vi "DriveToDistance.vi"() -> (0 "Drive Y Command":dbl format="%#_13g", 3 "Drive X Command":dbl format="%#_13g")   [LabVIEW 2016]
uses:
  Robot Global Data.vi
  <vilib>/addons/control/pid/pid.llb/PID Lead-Lag (DBL).vi
  <vilib>/addons/control/pid/pid.llb/PID (DBL).vi
  <vilib>/addons/control/pid/NI_PID_pid.lvlib
panel:
  in  "PID gains":T1={"proportional gain (Kc)"=0.05, "integral time (Ti, min)"=0.0, "derivative time (Td, min)"=0.0} {"derivative time (Td, min)" format="%.3f"; "integral time (Ti, min)" format="%.3f"; "proportional gain (Kc)" format="%.3f"}
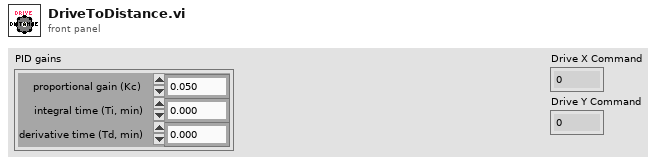
[diagram p1: front panel]
types:
  T1 = cluster{"proportional gain (Kc)":dbl, "integral time (Ti, min)":dbl, "derivative time (Td, min)":dbl}
  T2 = enum16{"FL Drive Wheel", "FR Drive Wheel", "RL Drive Wheel", "RR Drive Wheel", "FL Steer Wheel", "FR Steer Wheel", "RL Steer Wheel", "RR Steer Wheel"}
  T3 = typedef "WPI_MotorControlDeviceRef.ctl" = cluster{"DeviceStatus":errorcluster, "Type":T4, "PWM":cluster{"PWM Channel":T5, "DeadBand":T6}, "CAN":cluster{"Device Number":u8, "SetOutput VI Ref":variant, "GetOutput VI Ref":variant, "Enable VI Ref":variant, "Disable VI Ref":variant, "Data":variant}, "Invert":bool}
  T4 = typedef "WPI_MotorControlType.ctl" = enum16{"PWM", "CAN"}
  T5 = typedef "FPGA_DIOPWMChannel.ctl" = enum8{"PWM 0", "PWM 1", "PWM 2", "PWM 3", "PWM 4", "PWM 5", "PWM 6", "PWM 7", "PWM 8", "PWM 9", "PWM MXP 0", "PWM MXP 1", "PWM MXP 2", "PWM MXP 3", "PWM MXP 4", "PWM MXP 5", "PWM MXP 6", "PWM MXP 7", "PWM MXP 8", "PWM MXP 9", "Invalid"}
  T6 = typedef "WPI_PWMDeadband.ctl" = cluster{"Name":string, "maxPositivePwm":i32, "minPositivePwm":i32, "centerPwm":i32, "maxNegativePwm":i32, "minNegativePwm":i32, "angularRange":u16}
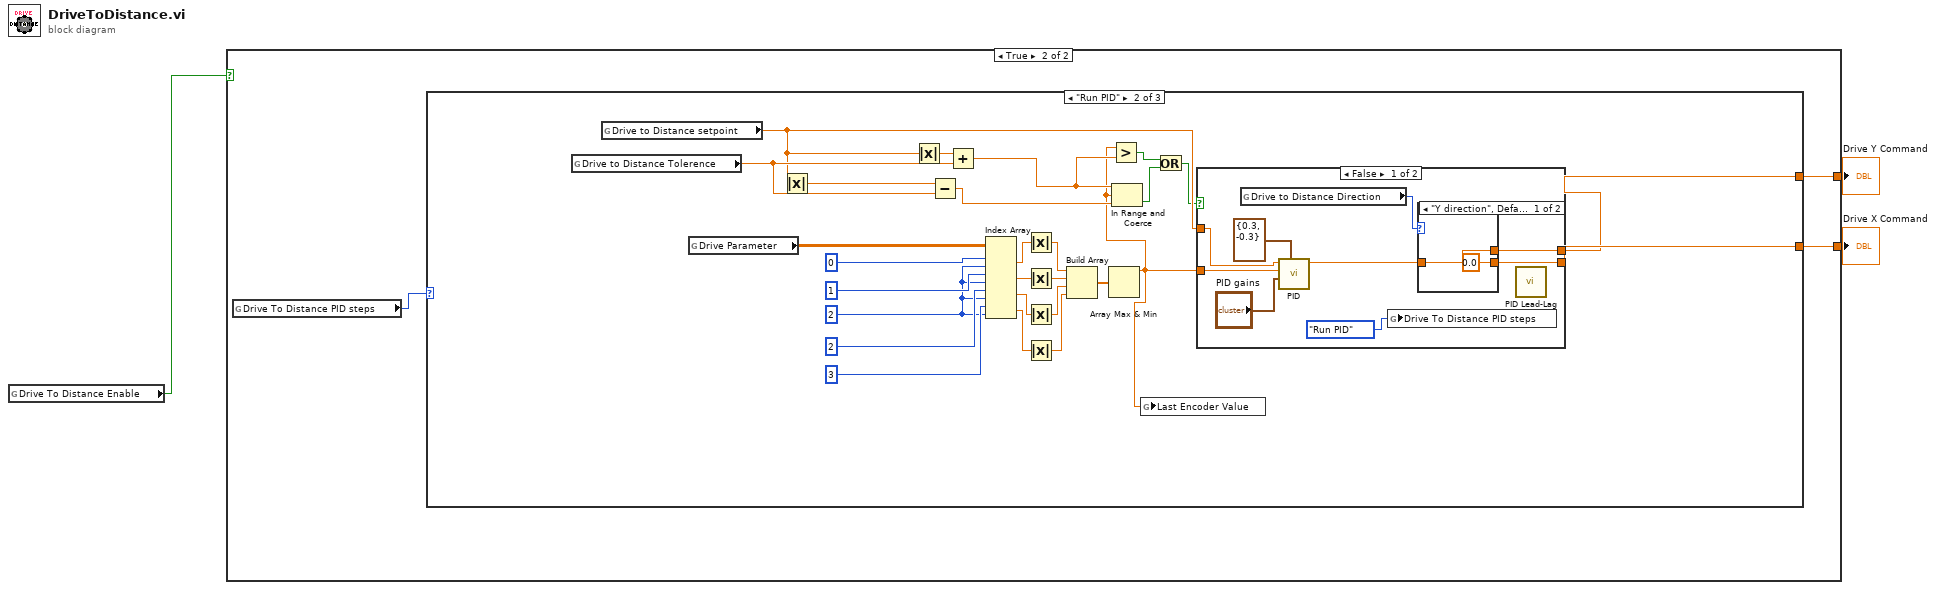
[diagram p0: block diagram]
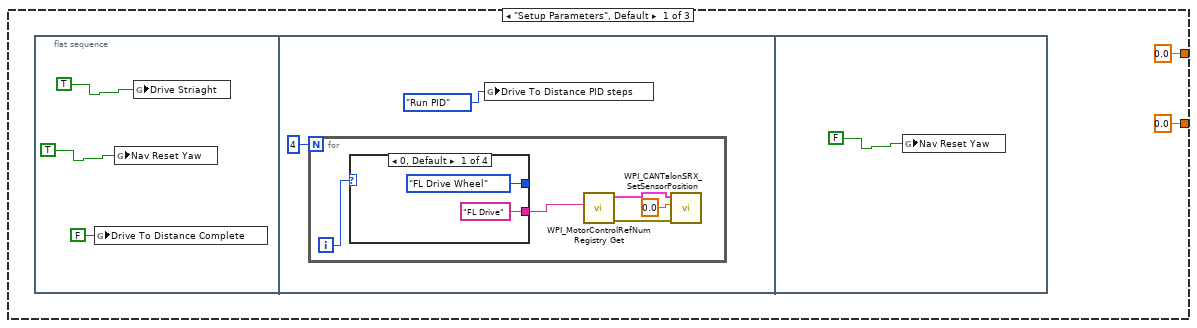
[diagram p3: hidden frame]
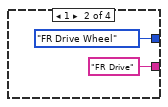
[diagram p4: hidden frame]
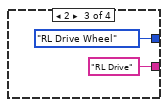
[diagram p5: hidden frame]
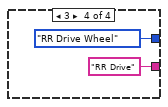
[diagram p6: hidden frame]
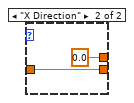
[diagram p7: hidden frame]
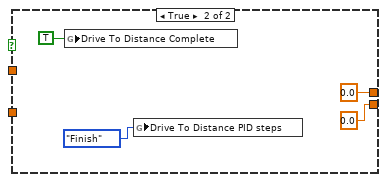
[diagram p8: hidden frame]
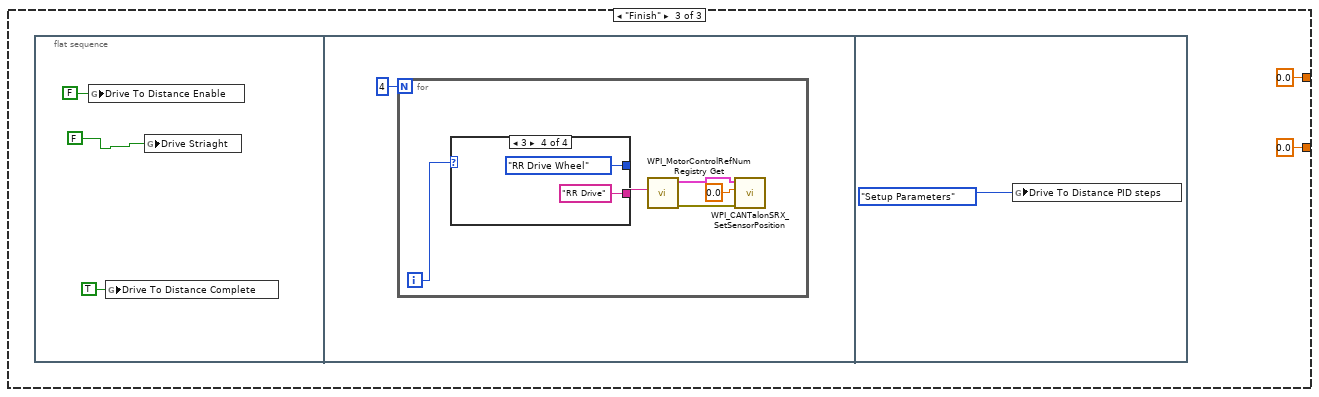
[diagram p9: hidden frame]
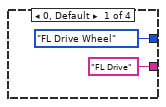
[diagram p10: hidden frame]
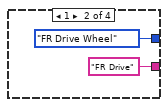
[diagram p11: hidden frame]
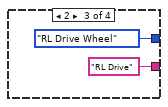
[diagram p12: hidden frame]
diagram:
  n1 = global read "Robot Global Data.vi" "Drive To Distance Enable"() -> (w3:bool)
  n2 = case shown="True" w3 {
    tunnel: [_ w6] -> w2
    tunnel: [_ w5] -> w1
    frame False {
    }
    frame True {
      n3 = global read "Robot Global Data.vi" "Drive To Distance PID steps"() -> (w4:enum16{"Setup Parameters", "Run PID", "Finish"})
      n4 = case shown="\"Run PID\"" w4 {
        tunnel: [0.0 ("Drive Command") w54 0.0 ("Drive Command")] -> w6
        tunnel: [0.0 ("output") w53 0.0 ("output")] -> w5
        frame "Setup Parameters", Default {
          n5 = flat-sequence {
            frame #0 {
              n6 = global write "Robot Global Data.vi" "Drive To Distance Complete"(FALSE ("Drive To Distance Complete")) -> ()
              n7 = global write "Robot Global Data.vi" "Nav Reset Yaw"(TRUE ("Drive Striaght")) -> ()
              n8 = global write "Robot Global Data.vi" "Drive Striaght"(TRUE ("Drive Striaght")) -> ()
            }
            frame #1 {
              n9 = for {
                N: 4 -> [_]
                i -> [w14]
                n10 = case shown="0, Default" w14 {
                  tunnel: [T2."FL Drive Wheel" ("Swerve Drive Param") T2."FR Drive Wheel" ("Swerve Drive Param") T2."RL Drive Wheel" ("Swerve Drive Param") T2."RR Drive Wheel" ("Swerve Drive Param")] -> _
                  tunnel: ["FL Drive" ("refnum name") "FR Drive" ("refnum name") "RL Drive" ("refnum name") "RR Drive" ("refnum name")] -> w18
                  frame 0, Default {
                  }
                  frame 1 {
                  }
                  frame 2 {
                  }
                  frame 3 {
                  }
                }
                n11 = call <vilib>:"WPI_MotorControlRefNum Registry Get.vi"("refnum name"=w18) -> ("error out"=w17:errorcluster, "MotorControlDevRef"=w16:T3)  [unwired: 9 in]
                n12 = call <vilib>:"WPI_CANTalonSRX_SetSensorPosition.vi"("error in (no error)"=w17, "New Sensor Position"=0.0, "CAN Talon SRX Ref"=w16) -> ()  [unwired: 7 in, 2 out]
              }
              n13 = global write "Robot Global Data.vi" "Drive To Distance PID steps"(enum16{"Setup Parameters", "Run PID", "Finish"}."Run PID" ("Drive To Distance PID steps")) -> ()
            }
            frame #2 {
              n14 = global write "Robot Global Data.vi" "Nav Reset Yaw"(FALSE ("Drive Striaght")) -> ()
            }
          }
        }
        frame "Run PID" {
          w47 = 2 ("disabled index (col)")
          n15 = global read "Robot Global Data.vi" "Drive to Distance Tolerence"() -> (w38:dbl)
          n16 = global read "Robot Global Data.vi" "Drive to Distance setpoint"() -> (w36:dbl)
          n17 = global read "Robot Global Data.vi" "Drive Parameter"() -> (w51:dbl[][])
          n18 = Absolute Value(x=w36) -> (abs(x)=w35:dbl)
          n19 = Absolute Value(x=w36) -> (abs(x)=w30:dbl)
          n20 = Subtract(x=w35, y=w38) -> (x-y=w34:dbl)
          n21 = Add(x=w30, y=w38) -> (x+y=w31:dbl)
          n22 = Index Array(array=w51, index (row) #1=0 ("index (row)"), index (col) #1=w47, index (row) #2=1 ("index (row)"), index (col) #2=w47, index (row) #3=2 ("index (row)"), index (col) #3=w47, index (row) #4=3 ("index (row)"), index (col) #4=w47) -> (element #1=w46:dbl, element #2=w45:dbl, element #3=w44:dbl, element #4=w43:dbl)
          n23 = Absolute Value(x=w46) -> (abs(x)=w37:dbl)
          n24 = Absolute Value(x=w45) -> (abs(x)=w40:dbl)
          n25 = Absolute Value(x=w44) -> (abs(x)=w41:dbl)
          n26 = Absolute Value(x=w43) -> (abs(x)=w42:dbl)
          n27 = Build Array(w37, w40, w41, w42) -> (w39:dbl[])
          n28 = Array Max & Min(array=w39) -> (max value=w28:dbl)  [unwired: 3 out]
          n29 = Greater?(x=w28, y=w31) -> (0:w32:bool)
          n30 = In Range and Coerce(upper limit=w31, x=w28, lower limit=w34) -> (In Range?=w33:bool)  [unwired: 1 out]
          n31 = global write "Robot Global Data.vi" "Last Encoder Value"(w28) -> ()
          n32 = Or(x=w32, y=w33) -> (x .or. y?=w29:bool)
          n33 = case shown="False" w29 {
            tunnel: w28 -> [w61 _]
            tunnel: w36 -> [w60 _]
            tunnel: [w57 0.0 ("Drive Command")] -> w54
            tunnel: [w56 0.0 ("output")] -> w53
            frame False {
              n34 = global read "Robot Global Data.vi" "Drive to Distance Direction"() -> (w59:enum16{"Y direction", "X Direction"})
              n35 = call-poly <vilib>:"PID.vi"("output range"=cluster{"output high":dbl, "output low":dbl} {"output high"=0.3, "output low"=-0.3}, "PID gains"="PID gains", "process variable"=w61, "setpoint"=w60) -> ("output"=w58:dbl)  [unwired: 6 in, 1 out]
              n36 = global write "Robot Global Data.vi" "Drive To Distance PID steps"(enum16{"Setup Parameters", "Run PID", "Finish"}."Run PID" ("Drive To Distance PID steps")) -> ()
              n37 = case shown="\"Y direction\", Default" w59 {
                tunnel: w58 -> [w64 w67]
                tunnel: [0.0 ("output") w67] -> w57
                tunnel: [w64 0.0 ("output")] -> w56
                frame "Y direction", Default {
                }
                frame "X Direction" {
                }
              }
              n38 = call-poly <vilib>:"PID Lead-Lag.vi"() -> ()  [unwired: 8 in, 2 out]
            }
            frame True {
              n39 = global write "Robot Global Data.vi" "Drive To Distance Complete"(TRUE ("Drive To Distance Complete")) -> ()
              n40 = global write "Robot Global Data.vi" "Drive To Distance PID steps"(enum16{"Setup Parameters", "Run PID", "Finish"}."Finish" ("Drive To Distance PID steps")) -> ()
            }
          }
        }
        frame "Finish" {
          n41 = flat-sequence {
            frame #0 {
              n42 = global write "Robot Global Data.vi" "Drive To Distance Enable"(FALSE ("Drive To Distance Enable")) -> ()
              n43 = global write "Robot Global Data.vi" "Drive To Distance Complete"(TRUE ("Drive To Distance Complete")) -> ()
              n44 = global write "Robot Global Data.vi" "Drive Striaght"(FALSE ("Drive Striaght")) -> ()
            }
            frame #1 {
              n45 = for {
                N: 4 -> [_]
                i -> [w78]
                n46 = case shown="3" w78 {
                  tunnel: [T2."FL Drive Wheel" ("Swerve Drive Param") T2."FR Drive Wheel" ("Swerve Drive Param") T2."RL Drive Wheel" ("Swerve Drive Param") T2."RR Drive Wheel" ("Swerve Drive Param")] -> _
                  tunnel: ["FL Drive" ("refnum name") "FR Drive" ("refnum name") "RL Drive" ("refnum name") "RR Drive" ("refnum name")] -> w79
                  frame 0, Default {
                  }
                  frame 1 {
                  }
                  frame 2 {
                  }
                  frame 3 {
                  }
                }
                n47 = call <vilib>:"WPI_MotorControlRefNum Registry Get.vi"("refnum name"=w79) -> ("error out"=w80:errorcluster, "MotorControlDevRef"=w81:T3)  [unwired: 9 in]
                n48 = call <vilib>:"WPI_CANTalonSRX_SetSensorPosition.vi"("error in (no error)"=w80, "New Sensor Position"=0.0, "CAN Talon SRX Ref"=w81) -> ()  [unwired: 7 in, 2 out]
              }
            }
            frame #2 {
              n49 = global write "Robot Global Data.vi" "Drive To Distance PID steps"(enum16{"Setup Parameters", "Run PID", "Finish"}."Setup Parameters" ("Drive To Distance PID steps")) -> ()
            }
          }
        }
      }
    }
  }
  "Drive X Command" <- w2
  "Drive Y Command" <- w1
